vi "Set API.vi"(8 "error in (no error)":errorcluster, 10 "Actor API":refnum<class "Actor API.lvclass">, 11 "Test 1 in":refnum<class "Test Caller.lvclass">) -> (0 "error out":errorcluster, 3 "Test 1 out":refnum<class "Test Caller.lvclass">)   [LabVIEW 2022 SP3, in "Scratchpad.lvlib" / "Test Caller.lvlib" / "Test Caller.lvclass"]
uses:
  Test Caller.lvclass
  Artifex/Actor Proxy/Actor API.lvclass
  Test Caller.lvclass/Test Caller.ctl
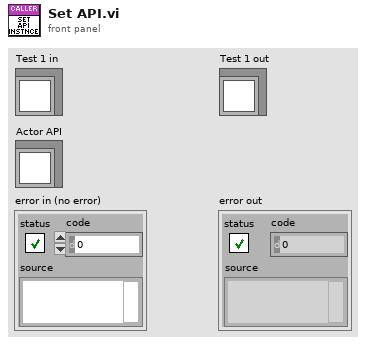
[diagram p1: front panel]
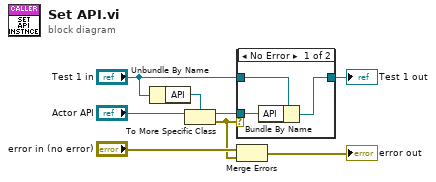
[diagram p0: block diagram]
diagram:
  n1 = Unbundle By Name("Test 1 in") -> ("API"=w6:refnum<class "Test Caller API.lvclass">)
  n2 = To More Specific Class(target class=w6, reference="Actor API") -> (specific class reference=w5:refnum<class "Test Caller API.lvclass">, error out=w1:errorcluster)  [unwired: 1 in]
  n3 = case shown="No Error" w1 {
    tunnel: w5 -> [w10 _]
    tunnel: "Test 1 in" -> [w11 w12]
    tunnel: [w9 w12] -> w3
    frame No Error {
      n4 = Bundle By Name(cluster=w11, "API"=w10) -> (w9:refnum<class "Test Caller.lvclass">)
    }
    frame Error {
    }
  }
  "Test 1 out" <- w3
  n5 = Merge Errors("error in (no error)", w1) -> (→"error out":errorcluster)
